vi "get_union.vi"(8 "error in (no error)":errorcluster, 11 "PositionSignals in":refnum<class "PositionSignals.lvclass">) -> (0 "error out":errorcluster, 3 "PositionSignals out":refnum<class "PositionSignals.lvclass">)   [LabVIEW 2010, in "PositionSignals.lvclass"]
uses:
  PositionSignals.lvclass
  PositionSignals.lvclass/PositionSignals.ctl
  common/classes/ImageCollection/ImageCollection/ImageCollection.lvclass
panel:
  out "union coordinates (x/y/z)":sgl[](array[numeric])
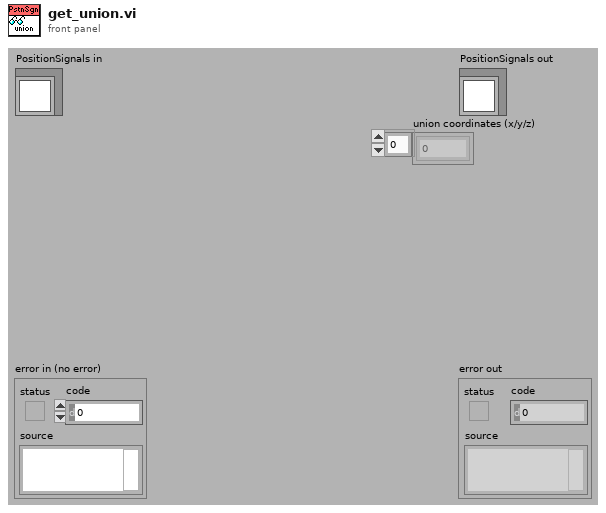
[diagram p1: front panel]
types:
  T1 = cluster{"x/y/z coordinates[0]":refnum<class "ImageCollection.lvclass">, "x/y/z coordinates[1]":refnum<class "ImageCollection.lvclass">, "x/y/z coordinates[2]":refnum<class "ImageCollection.lvclass">}
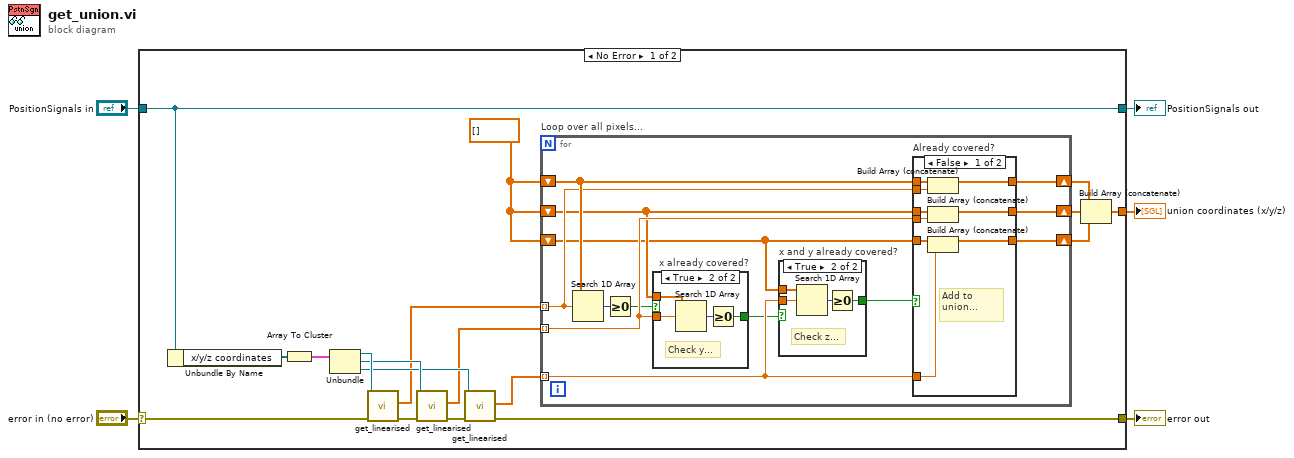
[diagram p0: block diagram]
diagram:
  n1 = case shown="No Error" "error in (no error)" {
    selector: "error in (no error)" -> [w18 w58]
    tunnel: [w22 w58] -> w4
    tunnel: [w23 w57] -> w2
    tunnel: "PositionSignals in" -> [w23 w57]
    tunnel: [w6 _] -> w1
    frame No Error {
      w10 = sgl[] []
      n2 = Unbundle By Name(w23) -> ("x/y/z coordinates"=w21:refnum<class "ImageCollection.lvclass">[])
      n3 = Array To Cluster(array=w21) -> (cluster=w20:T1)
      n4 = Unbundle(w20) -> ("x/y/z coordinates[0]"=w16:refnum<class "ImageCollection.lvclass">, "x/y/z coordinates[1]"=w15:refnum<class "ImageCollection.lvclass">, "x/y/z coordinates[2]"=w14:refnum<class "ImageCollection.lvclass">)
      n5 = call "get_linearised.vi"("error in (no error)"=w18, "ImageCollection in"=w16) -> ("error out"=w19:errorcluster, "pixels"=w13:sgl[])  [unwired: 7 in, 1 out]
      n6 = call "get_linearised.vi"("error in (no error)"=w19, "ImageCollection in"=w15) -> ("error out"=w17:errorcluster, "pixels"=w12:sgl[])  [unwired: 7 in, 1 out]
      n7 = call "get_linearised.vi"("error in (no error)"=w17, "ImageCollection in"=w14) -> ("error out"=w22:errorcluster, "pixels"=w11:sgl[])  [unwired: 7 in, 1 out]
      n8 = for "Loop over all pixels..." {
        tunnel: w13 -> [w35] mode=indexing
        tunnel: w12 -> [w31] mode=indexing
        tunnel: w11 -> [w27] mode=indexing
        shift-right: [w34] -> w9
        shift-left: w10 -> [w36]
        shift-right: [w33] -> w8
        shift-left: w10 -> [w30]
        shift-right: [w32] -> w7
        shift-left: w10 -> [w28]
        n9 = Search 1D Array(1D array=w36, element=w35) -> (index of element=w29:i32)  [unwired: 1 in]
        n10 = Greater Or Equal To 0?(x=w29) -> (x >= 0?=w26:bool)
        n11 = case "x already covered?" shown="True" w26 {
          tunnel: w31 -> [_ w56]
          tunnel: w30 -> [_ w55]
          tunnel: [_ w53] -> w25
          frame False {
          }
          frame True {
            # "Check y..."
            n12 = Search 1D Array(1D array=w55, element=w56) -> (index of element=w54:i32)  [unwired: 1 in]
            n13 = Greater Or Equal To 0?(x=w54) -> (x >= 0?=w53:bool)
          }
        }
        n14 = case "x and y already covered?" shown="True" w25 {
          tunnel: w28 -> [_ w51]
          tunnel: w27 -> [_ w50]
          tunnel: [_ w49] -> w24
          frame False {
          }
          frame True {
            # "Check z..."
            n15 = Search 1D Array(1D array=w51, element=w50) -> (index of element=w52:i32)  [unwired: 1 in]
            n16 = Greater Or Equal To 0?(x=w52) -> (x >= 0?=w49:bool)
          }
        }
        n17 = case "Already covered?" shown="False" w24 {
          tunnel: w36 -> [w45 w48]
          tunnel: w35 -> [w44 _]
          tunnel: [w43 w48] -> w34
          tunnel: [w42 w47] -> w33
          tunnel: [w41 w46] -> w32
          tunnel: w31 -> [w40 _]
          tunnel: w30 -> [w39 w47]
          tunnel: w28 -> [w38 w46]
          tunnel: w27 -> [w37 _]
          frame False {
            # "Add to union..."
            n18 = Build Array (concatenate)(w45, w44) -> (w43:sgl[])
            n19 = Build Array (concatenate)(w39, w40) -> (w42:sgl[])
            n20 = Build Array (concatenate)(w38, w37) -> (w41:sgl[])
          }
          frame True {
          }
        }
      }
      n21 = Build Array (concatenate)(w9, w8, w7) -> (w6:sgl[])
    }
    frame Error {
    }
  }
  "error out" <- w4
  "PositionSignals out" <- w2
  "union coordinates (x/y/z)" <- w1
